vi "[ModBus Ethernet Example Slave_32].vi"() -> ()   [LabVIEW 2010]
uses:
  MB Slave Init (poly).vi
  MB Globals.vi
  MB Slave Read All Coils (poly).vi
  MB Slave Read All Holding Registers (poly).vi
  MB Slave Write Input Registers (poly).vi
  MB Slave Write Discrete Inputs (poly).vi
panel:
  in  "Discrete Inputs (Read only)":bool[](array[boolean])=[FALSE, FALSE, FALSE, FALSE, FALSE, FALSE, FALSE, FALSE, FALSE, FALSE, FALSE, FALSE, FALSE, FALSE, FALSE, FALSE, FALSE, FALSE, FALSE, FALSE, FALSE, FALSE, FALSE, FALSE, FALSE, FALSE, FALSE, FALSE, TRUE, TRUE]
  in  "Input Registers (Read Only)":sgl[](array[numeric])=[0.0, 0.0, 0.0, 0.0]
  in  "TCP服务端口":u16=502
  in  "Stop":bool
  out "Holding Registers":sgl[](array[numeric]) caption="Holding Registers (Read&Write)"
  out "Coils":bool[](array[boolean]) caption="Coils (Master can write coils)"
  # "TCP Settings"
  # "Slave Registers"
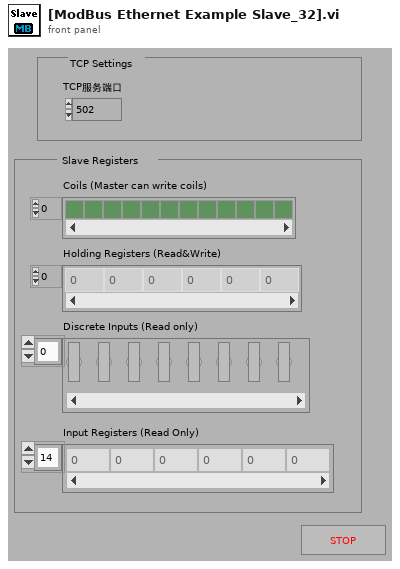
[diagram p1: front panel]
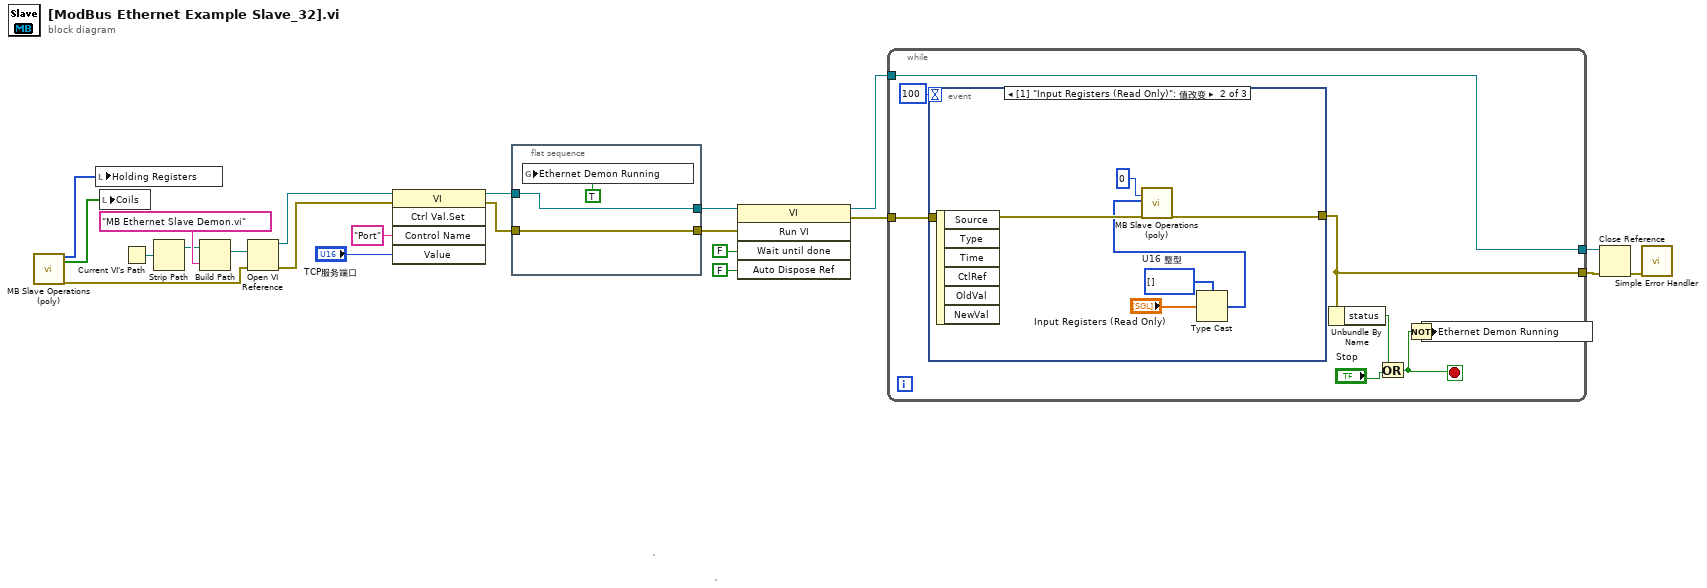
[diagram p0: block diagram]
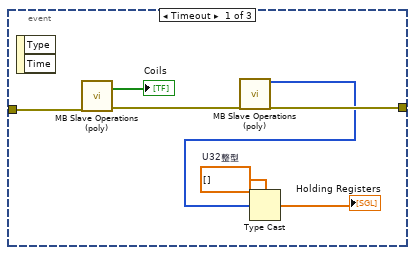
[diagram p2: hidden frame]
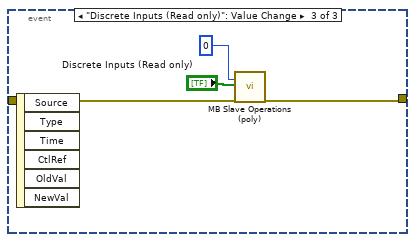
[diagram p3: hidden frame]
diagram:
  n1 = call-poly "MB Slave Operations (poly).vi"() -> ("Holding Registers"=w22:u16[], "Coils"=w6:bool[], "error out"=w9:errorcluster)  [unwired: 1 in, 16 out]
  n2 = local write "Holding Registers"(w22) -> ()
  n3 = local write "Coils"(w6) -> ()
  n4 = Current VI's Path() -> (path=w18:path)
  n5 = Strip Path(path=w18) -> (stripped path=w19:path)  [unwired: 1 out]
  n6 = Build Path(base path=w19, name or relative path="MB Ethernet Slave Demon.vi") -> (appended path=w21:path)
  n7 = Open VI Reference(vi path=w21, error in (no error)=w9) -> (vi reference=w15:refnum<vi>, error out=w14:errorcluster)  [unwired: 4 out]
  n8 = invoke class="VI" method="Ctrl Val.Set"(reference=w15, error in=w14, "Control Name"="Port", "Value"="TCP服务端口") -> (reference out=w2:refnum<vi>, error out=w3:errorcluster)  [unwired: 1 in, 3 out]
  n9 = flat-sequence {
    tunnel: [w25] -> w8
    tunnel: w3 -> [w25]
    tunnel: [w23] -> w5
    tunnel: w2 -> [w23]
    frame #0 {
      n10 = global write "MB Globals.vi" "Ethernet Demon Running"(TRUE ("Slave Demon Running")) -> ()
    }
  }
  n11 = invoke class="VI" method="Run VI"(reference=w5, error in=w8, "Wait until done"=FALSE, "Auto Dispose Ref"=FALSE) -> (reference out=w11:refnum<vi>, error out=w7:errorcluster)  [unwired: 1 in, 3 out]
  n12 = while {
    tunnel: [w28] -> w12
    tunnel: w11 -> [w28]
    tunnel: [w27] -> w10
    tunnel: w7 -> [w26]
    stop <- w29 stop-if-true
    n13 = event shown="[1] \"Input Registers (Read Only)\": 值改变" {
      selector: _ -> [_ _ _]
      dyn-events: _ -> [_ _ _]
      timeout: 100 -> [_ _ _]
      tunnel: w26 -> [w40 w46 w50]
      tunnel: [w37 w44 w48] -> w27
      event Timeout {
        w36 = sgl[] []  # U32整型
        n14 = event-data() -> ()  [unwired: 3 out]
        n15 = call-poly "MB Slave Operations (poly).vi"("error in"=w40) -> ("Coils"=→"Coils":bool[], "error out"=w38:errorcluster)  [unwired: 17 out]
        n16 = call-poly "MB Slave Operations (poly).vi"("error in"=w38) -> ("Holding Registers"=w35:u16[], "error out"=w37:errorcluster)  [unwired: 17 out]
        n17 = Type Cast(type=w36, x=w35) -> (*(type *) &x=→"Holding Registers":sgl[])
      }
      event "Input Registers (Read Only)": Value Change {
        w43 = u16[] []  # U16 整型
        n18 = event-data() -> ()  [unwired: 7 out]
        n19 = Type Cast(type=w43, x="Input Registers (Read Only)") -> (*(type *) &x=w41:u16[])
        n20 = call-poly "MB Slave Operations (poly).vi"("Starting Address"=u16 0 ("Address"), "Input Registers"=w41, "error in"=w46) -> ("error out"=w44:errorcluster)  [unwired: 1 in, 15 out]
      }
      event "Discrete Inputs (Read only)": Value Change {
        n21 = event-data() -> ()  [unwired: 7 out]
        n22 = call-poly "MB Slave Operations (poly).vi"("Starting Address"=u16 0, "Discrete Inputs"="Discrete Inputs (Read only)", "error in"=w50) -> ("error out"=w48:errorcluster)  [unwired: 1 in, 15 out]
      }
    }
    n23 = Unbundle By Name(w27) -> ("status"=w32:bool)
    n24 = Or(x=w32, y="Stop") -> (x .or. y?=w29:bool)
    n25 = Not(x=w29) -> (.not. x?=w30:bool)
    n26 = global write "MB Globals.vi" "Ethernet Demon Running"(w30) -> ()
  }
  n27 = Close Reference(reference=w12, error in (no error)=w10) -> (error out=w4:errorcluster)
  n28 = call <vilib>:"Simple Error Handler.vi"("error in (no error)"=w4) -> ()  [unwired: 1 in, 8 out]
